vi "oa_FIR Filter Based Sample Rate Conversion (Continuous) (1 channel).vi"(0 "even angle signal in":cluster{"r0":dbl, "dr":dbl, "Y":dbl[]}={"r0"=0.0, "dr"=1.0, "Y"=[]} {"r0" format="%.2p"; "dr" format="%.2p"; "Y" format="%.2f"}, 1 "reset? (T)":bool=TRUE, 5 "dr":dbl=1.0 format="%.2p", 7 "even angle position info":T1, 9 "FIR filter specifications":T2={"alias rejection (dB)"=120.0, "normalized bandwidth"=0.4536} {"normalized bandwidth" format="%.4f"; "alias rejection (dB)" format="%.2f"}, 11 "error in (no error)":errorcluster) -> (4 "even angle signal out":cluster{"r0":dbl, "dr":dbl, "Y":dbl[]}={"r0"=0.0, "dr"=1.0, "Y"=[]} {"r0" format="%.2p"; "dr" format="%.2p"; "Y" format="%.2f"}, 6 "even angle position info out":T1, 15 "error out":errorcluster)   [LabVIEW 2017, in "SoundVib_OAUtility.lvlib"]
uses:
  <vilib>/addons/Sound and Vibration/Order Analysis/Utility/SoundVib_OAUtility.lvlib
  <vilib>/addons/Sound and Vibration/Order Analysis/Misc/OAT Position Info.ctl
  <vilib>/measure/maresamp.llb/Resample Waveform (continuous, t0 DBL).vi
  <vilib>/measure/NI_MAPro.lvlib
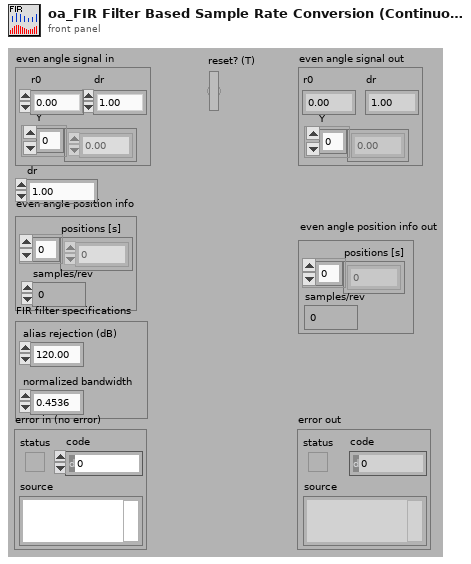
[diagram p1: front panel]
types:
  T1 = typedef "OAT Position Info.ctl" = cluster{"positions [s]":dbl[], "samples/rev":dbl}
  T2 = cluster{"alias rejection (dB)":dbl, "normalized bandwidth":dbl}
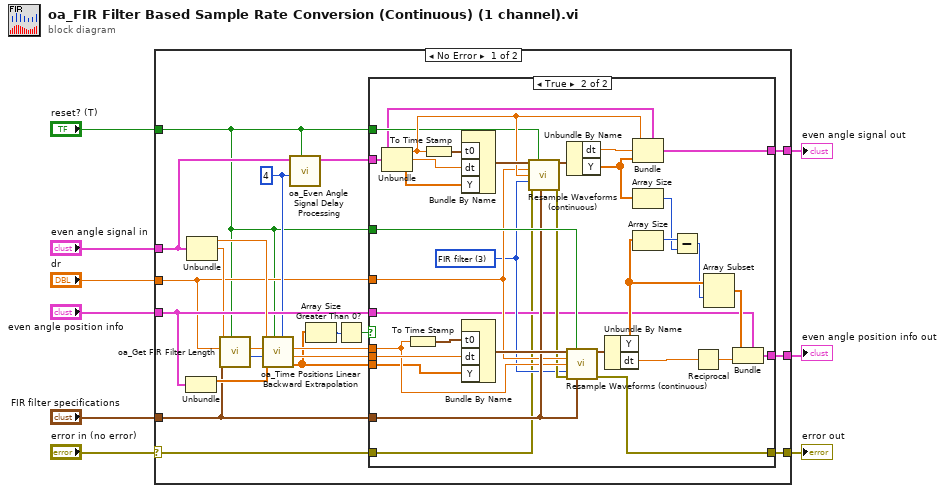
[diagram p0: block diagram]
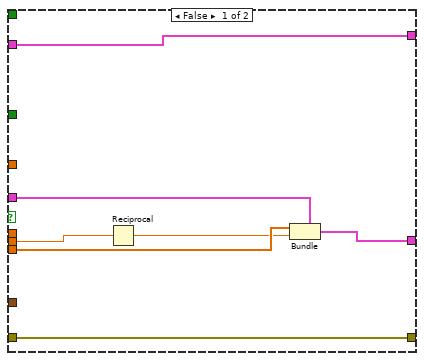
[diagram p2: hidden frame]
diagram:
  n1 = case shown="No Error" "error in (no error)" {
    selector: "error in (no error)" -> [w10 w73]
    tunnel: "even angle position info" -> [w28 w72]
    tunnel: [w27 w72] -> w8
    tunnel: "FIR filter specifications" -> [w25 _]
    tunnel: "even angle signal in" -> [w24 w71]
    tunnel: [w23 w71] -> w5
    tunnel: "dr" -> [w18 _]
    tunnel: [w14 w73] -> w3
    tunnel: "reset? (T)" -> [w11 _]
    frame No Error {
      w22 = 4 ("number of points")
      n2 = Unbundle(w28) -> ("positions [s]"=w30:dbl[])  [unwired: 1 out]
      n3 = Unbundle(w24) -> ("r0"=w29:dbl, "dr"=w21:dbl)  [unwired: 1 out]
      n4 = call <vilib>:"oa_Get FIR Filter Length.vi"("reset? (T)"=w11, "FIR filter specifications"=w25, "dr new"=w18, "dr old"=w21) -> ("filter length"=w20:i32, "dr old out"=w19:dbl)  [unwired: 6 in]
      n5 = call <vilib>:"oa_Time Positions Linear Backward Extrapolation.vi"("number of points"=w22, "reset? (T)"=w11, "positions [s]"=w30, "filter length"=w20, "dr"=w19, "r0"=w29) -> ("extraploated positions [s]"=w12:dbl[], "dr out"=w17:dbl, "new r0"=w16:dbl)  [unwired: 3 in]
      n6 = call <vilib>:"oa_Even Angle Signal Delay Processing.vi"("reset? (T)"=w11, "number of points"=w22, "even angle signal in"=w24) -> ("buffered even angle signal"=w26:cluster{"r0":dbl, "dr":dbl, "Y":dbl[]})  [unwired: 8 in]
      n7 = Array Size(array=w12) -> (size(s)=w15:i32)
      n8 = Greater Than 0?(x=w15) -> (x > 0?=w13:bool)
      n9 = case shown="True" w13 {
        tunnel: w11 -> [_ w68]
        tunnel: w28 -> [w36 w40]
        tunnel: [w35 w64] -> w27
        tunnel: w26 -> [w37 w38]
        tunnel: w25 -> [_ w59]
        tunnel: [w37 w55] -> w23
        tunnel: w18 -> [_ w54]
        tunnel: w17 -> [w33 w53]
        tunnel: w16 -> [_ w52]
        tunnel: w12 -> [w34 w51]
        tunnel: [w31 w48] -> w14
        tunnel: w11 -> [_ w47]
        tunnel: w10 -> [w31 w39]
        frame False {
          n10 = Reciprocal(x=w33) -> (1/x=w32:dbl)
          n11 = Bundle(cluster=w36, "positions [s]"=w34, "samples/rev"=w32) -> (w35:T1)
        }
        frame True {
          w49 = u16 3 items=["coerce", "linear", "spline", "FIR filter"] ("interpolation mode")
          n12 = Unbundle(w38) -> ("r0"=w56:dbl, "dr"=w62:dbl, "Y"=w63:dbl[])
          n13 = To Time Stamp(1:w52) -> (0:w69:timestamp)
          n14 = To Time Stamp(1:w56) -> (0:w61:timestamp)
          n15 = Bundle By Name("t0"=w61, "dt"=w62, "Y"=w63) -> (w60:waveform(dbl))  [unwired: 1 in]
          n16 = Bundle By Name("t0"=w69, "dt"=w53, "Y"=w51) -> (w70:waveform(dbl))  [unwired: 1 in]
          n17 = call-poly <vilib>:"Resample Waveforms (continuous).vi"("waveform in"=w60, "reset"=w47, "dt"=w54, "t0"=w56, "interpolation mode"=w49, "error in (no error)"=w39, "FIR filter specifications"=w59) -> ("resampled waveform out"=w58:waveform(dbl), "error out"=w50:errorcluster)  [unwired: 4 in, 3 out]
          n18 = Unbundle By Name(w58) -> ("dt"=w57:dbl, "Y"=w46:dbl[])
          n19 = call-poly <vilib>:"Resample Waveforms (continuous).vi"("waveform in"=w70, "reset"=w68, "dt"=w54, "t0"=w52, "interpolation mode"=w49, "error in (no error)"=w50, "FIR filter specifications"=w59) -> ("resampled waveform out"=w67:waveform(dbl), "error out"=w48:errorcluster)  [unwired: 4 in, 3 out]
          n20 = Unbundle By Name(w67) -> ("Y"=w42:dbl[], "dt"=w66:dbl)
          n21 = Bundle(cluster=w38, "r0"=w56, "dr"=w57, "Y"=w46) -> (w55:cluster{"r0":dbl, "dr":dbl, "Y":dbl[]})
          n22 = Array Size(array=w46) -> (size(s)=w44:i32)
          n23 = Array Size(array=w42) -> (size(s)=w45:i32)
          n24 = Subtract(x=w45, y=w44) -> (x-y=w41:i32)
          n25 = Reciprocal(x=w66) -> (1/x=w65:dbl)
          n26 = Array Subset(array=w42, index=w41) -> (w43:dbl[])  [unwired: 1 in]
          n27 = Bundle(cluster=w40, "positions [s]"=w43, "samples/rev"=w65) -> (w64:T1)
        }
      }
    }
    frame Error {
    }
  }
  "even angle signal out" <- w5
  "even angle position info out" <- w8
  "error out" <- w3
